vi "AddHelper.vi"() -> ()   [LabVIEW 2024, in "AddHelper.lvlib"]
uses:
  AddHelper.lvlib
  <vilib>/Utility/miscctls.llb/LVPointTypeDef.ctl
  <vilib>/Utility/traverseref.llb/TRef TravTarget.ctl
  <vilib>/event_ctls.llb/lveventtype.ctl
  templates/TemplateModule/TemplateModule.Start.vi
  templates/HelperTemplate.vi
  templates/TemplateModule/TemplateModule.lvclass
  <vilib>/Utility/traverseref.llb/VI Scripting - Traverse.lvlib
  <vilib>/Utility/Data Type/NI_Data Type.lvlib
panel:
  out "# of Refs 2":i32
  out "# of Refs":i32
  in  "Helper Name":string
  out "Child Type":refnum<vi>[](array[refnum])
  out "Same Type":refnum<vi>[](array[refnum])
  out "error out 2":errorcluster
  in  "Module Name":string
  out "Bottom":i32
  out "Left":i32
  out "error out":errorcluster
  in  "error in (no error)":errorcluster
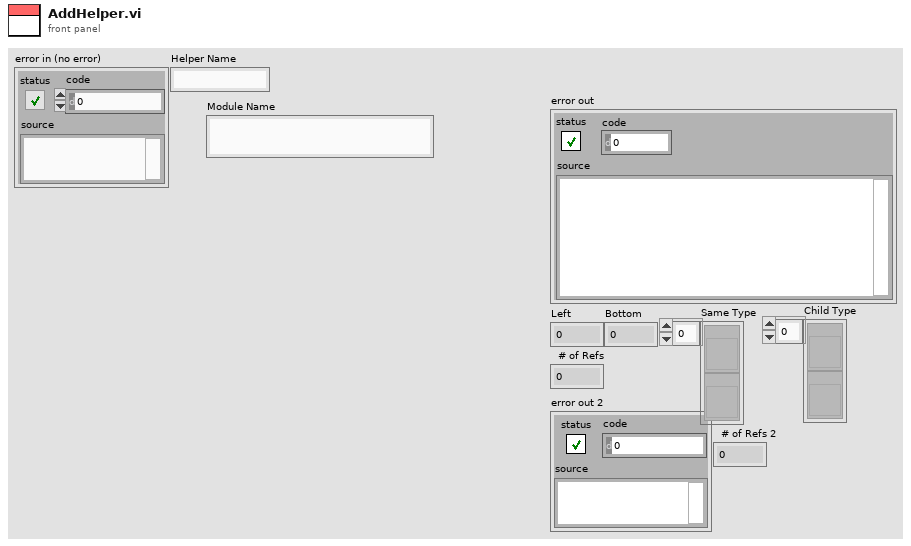
[diagram p1: front panel]
types:
  T1 = typedef "lveventtype.ctl" = enum32{"Null", "Timeout", "Annotation Menu Selection", "Annotation Menu Selection?", "App Instance Close", "App Instance Close?", "Autoscale Range Change", "Bookmark Info Change", "Cell Edit", "Cell Edit?", "Cursor Grab", "Cursor Grab?", "Cursor Menu Selection", "Cursor Menu Selection?", "Cursor Move", "Cursor Release", "Data Change", "Direction Change", "Display State Change", "Drag Ended", "Drag Enter", "Drag Leave", "Drag Over", "Drag Source Update", "Drag Starting", "Drag Starting?", "Drop", "Exec State Change", "Key Down", "Key Down?", "Key Repeat", "Key Repeat?", "Key Up", "Listbox Double Click", "Menu Activation?", "Menu Selection (App)", "Menu Selection? (App)", "Menu Selection (User)", "Mouse Down", "Mouse Down?", "Mouse Enter", "Mouse Leave", "Mouse Move", "Mouse Up", "Mouse Wheel", "NI Security User Change (App)", "Pane Size", "Panel Close", "Panel Close?", "Panel Resize", "Plot Attribute Change", "Scale Range Change", "Shortcut Menu Activation?", "Shortcut Menu Selection (App)", "Shortcut Menu Selection? (App)", "Shortcut Menu Selection (User)", "Tree Double Click", "Tree Drag", "Tree Drag?", "Tree Drop", "Tree Drop?", "Tree Item Close", "Tree Item Close?", "Tree Item Open", "Tree Item Open?", "User Event", "Value Change"}
  T2 = cluster{"Event Type":T1, "Event Registration Index":i32}[]
  T3 = typedef "TRef TravTarget.ctl" = enum16{"FP", "BD", "Other"}
  T4 = typedef "LVPointTypeDef.ctl" = cluster{"Horizontal":i16, "Vertical":i16}
  T5 = typedef "LVPositionTypeDef.ctl" = cluster{"Left":i32, "Top":i32}
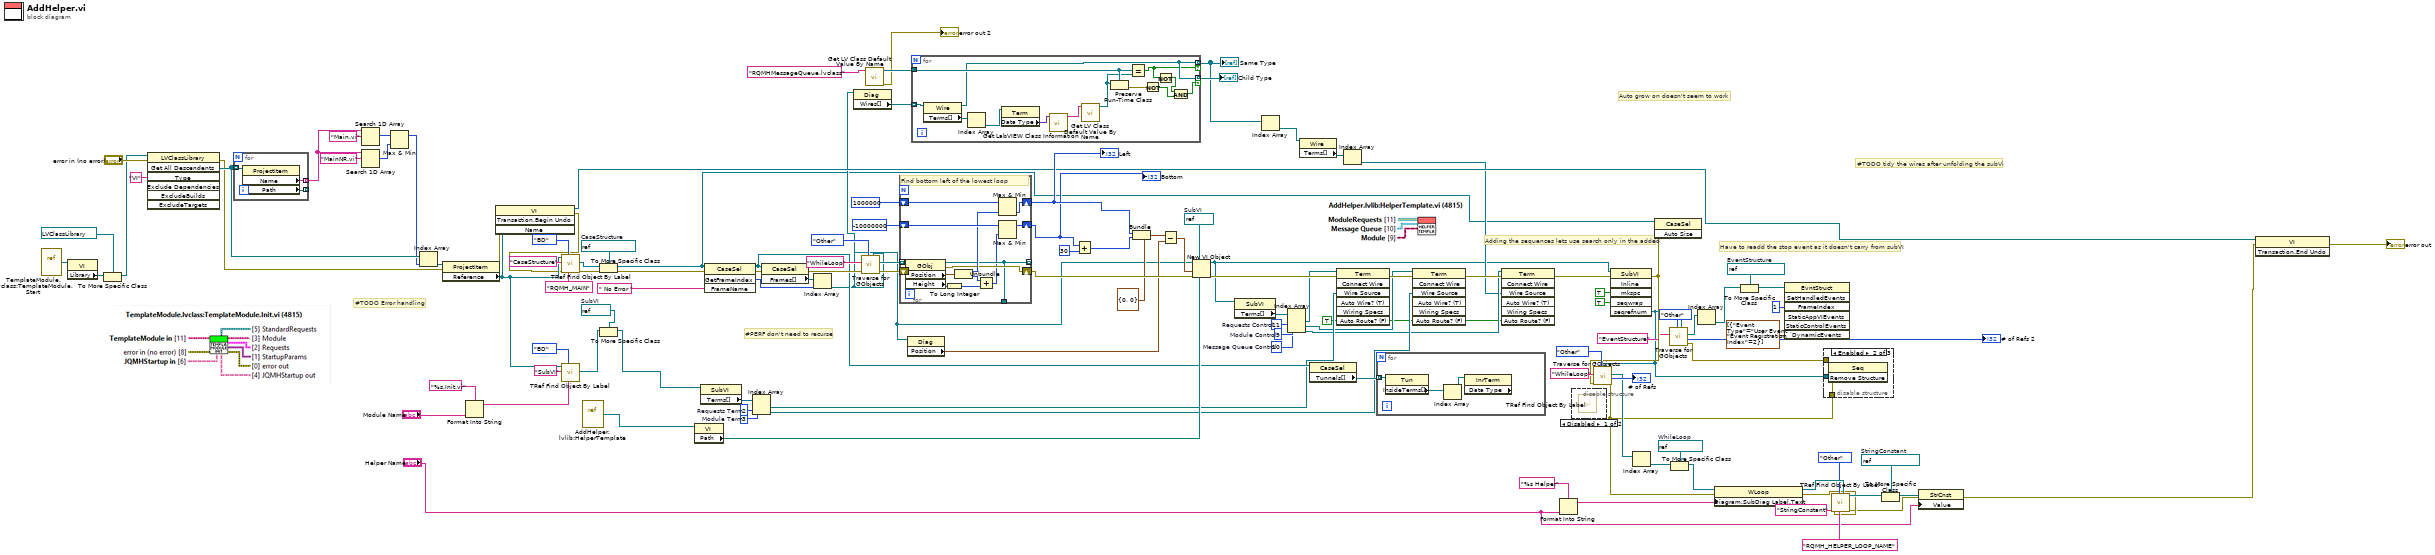
[diagram p0: block diagram]
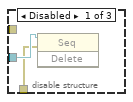
[diagram p2: hidden frame]
diagram:
  w7 = refnum<vi> refnum  # EventStructure
  w19 = refnum<vi> refnum  # StringConstant
  w30 = refnum<vi> refnum  # WhileLoop
  w58 = 10  # Message Queue Control
  w40 = TRUE ("Auto Route? (F)")
  w61 = 9  # Module Control
  w65 = 11  # Requests Control
  w67 = 3  # Module Term
  w68 = 2  # Requests Term
  w70 = refnum<vi> refnum  # SubVI
  w91 = refnum<vi> refnum  # SubVI
  w104 = refnum<vi> refnum  # CaseStructure
  # "Have to readd the stop event as it doesn't carry from subVI"
  # "#TODO tidy the wires after unfolding the subVi"
  # "Adding the sequences lets use search only in the added"
  # "Auto grow on doesn't seem to work"
  # "#PERF don't need to recurse"
  # "#TODO Error handling"
  n1 = vi-ref "TemplateModule.lvclass:TemplateModule.Start.vi"() -> (w110:refnum<vi>)
  n2 = property class="VI"(reference=w110) -> ("Library"=w108:refnum<vi>)  [unwired: 1 in, 2 out]
  n3 = To More Specific Class(target class=refnum<vi> refnum ("reference"), reference=w108) -> (specific class reference=w107:refnum<vi>)  [unwired: 1 in, 1 out]
  n4 = invoke class="LVClassLibrary" method="Get All Descendents"(reference=w107, error in="error in (no error)", "Type"="VI") -> (error out=w115:errorcluster, "All Descendents"=w118:refnum<vi>[])  [unwired: 4 in, 5 out]
  n5 = for {
    tunnel: w118 -> [w127] mode=indexing
    tunnel: [w126] -> w119 mode=indexing
    tunnel: [w125] -> _ mode=indexing
    n6 = property class="ProjectItem"(reference=w127) -> ("Name"=w126:string, "Path"=w125:path)  [unwired: 1 in, 2 out]
  }
  n7 = Search 1D Array(1D array=w119, element="Main.vi") -> (index of element=w121:i32)  [unwired: 1 in]
  n8 = Search 1D Array(1D array=w119, element="MainNR.vi") -> (index of element=w120:i32)  [unwired: 1 in]
  n9 = Max & Min(x=w121, y=w120) -> (max(x,y)=w116:i32)  [unwired: 1 out]
  n10 = Index Array(array=w118, index=w116) -> (element=w117:refnum<vi>)
  n11 = property class="ProjectItem"(reference=w117, error in=w115) -> (error out=w51:errorcluster, "Reference"=w52:refnum<vi>)  [unwired: 1 out]
  n12 = Format Into String(format string="%s.Init.vi", "Module Name") -> (resulting string=w75:string)  [unwired: 2 in, 1 out]
  n13 = invoke class="VI" method="Transaction.Begin Undo"(reference=w52, error in=w51) -> (reference out=w49:refnum<vi>, error out=w50:errorcluster)  [unwired: 2 in, 2 out]
  n14 = call <vilib>:"TRef Find Object By Label.vi"("Label"="RQMH_MAIN", "Traverse Target"=TRef_TravTarget."BD", "error in (no error)"=w50, "Class Name"="CaseStructure", "VI Ref"=w52) -> ("error out"=w106:errorcluster, "Found Obj Ref"=w105:refnum<vi>)  [unwired: 3 in, 2 out]
  n15 = call <vilib>:"TRef Find Object By Label.vi"("Label"=w75, "Traverse Target"=TRef_TravTarget."BD", "Class Name"="SubVI", "VI Ref"=w52) -> ("Found Obj Ref"=w72:refnum<vi>)  [unwired: 4 in, 3 out]
  n16 = vi-ref "AddHelper.lvlib:HelperTemplate.vi"() -> (w82:refnum<vi>)
  n17 = To More Specific Class(target class=w104, reference=w105, error in=w106) -> (specific class reference=w36:refnum<vi>, error out=w35:errorcluster)
  n18 = To More Specific Class(target class=w70, reference=w72) -> (specific class reference=w71:refnum<vi>)  [unwired: 1 in, 1 out]
  n19 = property class="VI"(reference=w82) -> ("Path"=w81:path)  [unwired: 1 in, 2 out]
  n20 = property class="SubVI"(reference=w71) -> ("Terms[]"=w69:refnum<vi>[])  [unwired: 1 in, 2 out]
  n21 = invoke class="CaseSel" method="GetFrameIndex"(reference=w36, error in=w35, "FrameName"=" No Error " ("Frame Name")) -> (reference out=w79:refnum<vi>, error out=w102:errorcluster, "GetFrameIndex"=w100:i32)  [unwired: 1 in, 1 out]
  n22 = Index Array(array=w69, index #1=w68, index #2=w67) -> (element #1=w63:refnum<vi>, element #2=w59:refnum<vi>)
  n23 = property class="CaseSel"(reference=w79, error in=w102) -> (error out=w99:errorcluster, "Frames[]"=w101:refnum<vi>[])  [unwired: 1 out]
  n24 = Index Array(array=w101, index=w100) -> (element=w47:refnum<vi>)
  n25 = property class="Diag"(reference=w47) -> ("Wires[]"=w46:refnum<vi>[])  [unwired: 1 in, 2 out]
  n26 = call <vilib>:"Traverse for GObjects.vi"("Other Refnum"=w47, "Traverse Target"=TRef_TravTarget."Other", "error in (no error)"=w99, "Class Name"="WhileLoop") -> ("error out"=w93:errorcluster, "References"=w96:refnum<vi>[])  [unwired: 4 in, 2 out]
  n27 = call <vilib>:"Get LV Class Default Value By Name.vi"("class name"="RQMHMessageQueue.lvclass") -> ("error out"=→"error out 2":errorcluster, "object"=w44:refnum<class>)  [unwired: 9 in]
  n28 = for {
    tunnel: w96 -> [w141] mode=indexing
    tunnel: [w133] -> _ mode=indexing
    shift-right: [w137] -> w86
    shift-left: 1000000 ("Left") -> [w139]
    shift-right: [w132] -> w85
    shift-left: -10000000 ("Left") -> [w138]
    shift-right: [w134] -> w92
    shift-left: w93 -> [w135]
    tunnel: [w133] -> _
    # "Find bottom left of the lowest loop"
    n29 = property class="GObj"(reference=w141, error in=w135) -> (reference out=w133:refnum<vi>, error out=w134:errorcluster, "Position"=w140:T5, "Height"=w130:u32)
    n30 = To Long Integer(number=w130) -> (32bit integer=w128:i32)
    n31 = Unbundle(w140) -> ("Left"=w136:i32, "Top"=w131:i32)
    n32 = Add(x=w131, y=w128) -> (x+y=w129:i32)
    n33 = Max & Min(x=w139, y=w136) -> (min(x,y)=w137:i32)  [unwired: 1 out]
    n34 = Max & Min(x=w138, y=w129) -> (max(x,y)=w132:i32)  [unwired: 1 out]
  }
  "Left" <- w86
  "Bottom" <- w85
  n35 = property class="Diag"(reference=w47) -> ("Position"=w88:T5)  [unwired: 1 in, 2 out]
  n36 = for {
    tunnel: w46 -> [w154] mode=indexing
    tunnel: w44 -> [w148]
    tunnel: [w146] -> w41 mode=indexing if=w145
    tunnel: [w146] -> w42 mode=indexing if=w142
    n37 = property class="Wire"(reference=w154) -> (reference out=w146:refnum<vi>, "Terms[]"=w153:refnum<vi>[])  [unwired: 1 in, 1 out]
    n38 = Index Array(array=w153) -> (element=w152:refnum<vi>)  [unwired: 1 in]
    n39 = property class="Term"(reference=w152) -> ("Data Type"=w151:variant)  [unwired: 1 in, 2 out]
    n40 = call <vilib>:"Get LabVIEW Class Information.vi"("variant"=w151) -> ("LabVIEW class file name"=w150:string)  [unwired: 8 in, 2 out]
    n41 = call <vilib>:"Get LV Class Default Value By Name.vi"("class name"=w150) -> ("object"=w147:refnum<class>)  [unwired: 9 in, 1 out]
    n42 = Preserve Run-Time Class(object in=w147, 2:w148) -> (error out=w149:errorcluster)  [unwired: 1 in, 1 out]
    n43 = Equal?(x=w148, y=w147) -> (x = y?=w145:bool)
    n44 = Not(x=w149) -> (.not. x?=w144:bool)
    n45 = Not(x=w145) -> (.not. x?=w143:bool)
    n46 = And(x=w143, y=w144) -> (x .and. y?=w142:bool)
  }
  "Same Type" <- w41
  "Child Type" <- w42
  n47 = Add(x=w85, y=30) -> (x+y=w83:i32)
  n48 = Bundle(cluster=T4 {"Horizontal"=0, "Vertical"=0} ("location"), "Horizontal"=w86, "Vertical"=w83) -> (w89:T4)
  n49 = Subtract(x=w89, y=w88) -> (x-y=w87:T5)
  n50 = New VI Object(vi object class=w91, owner refnum=w47, position/next to=w87, 6:w81, 8:w92) -> (object refnum=w34:refnum<vi>, 0:w80:errorcluster)  [unwired: 3 in]
  n51 = property class="SubVI"(reference=w34) -> ("Terms[]"=w66:refnum<vi>[])  [unwired: 1 in, 2 out]
  n52 = Index Array(array=w41) -> (element=w38:refnum<vi>)  [unwired: 1 in]
  n53 = Index Array(array=w66, index #1=w65, index #2=w61, index #3=w58) -> (element #1=w64:refnum<vi>, element #2=w60:refnum<vi>, element #3=w54:refnum<vi>)
  n54 = property class="Wire"(reference=w38) -> ("Terms[]"=w39:refnum<vi>[])  [unwired: 1 in, 2 out]
  n55 = property class="CaseSel"(reference=w79) -> ("Tunnels[]"=w78:refnum<vi>[])  [unwired: 1 in, 2 out]
  n56 = invoke class="Term" method="Connect Wire"(reference=w64, error in=w80, "Wire Source"=w63, "Auto Route? (F)"=w40) -> (error out=w62:errorcluster)  [unwired: 3 in, 6 out]
  n57 = Index Array(array=w39) -> (element=w37:refnum<vi>)  [unwired: 1 in]
  n58 = for {
    tunnel: w78 -> [w157] mode=indexing
    n59 = property class="Tun"(reference=w157) -> ("InsideTerms[]"=w156:refnum<vi>[])  [unwired: 1 in, 2 out]
    n60 = Index Array(array=w156) -> (element=w155:refnum<vi>)  [unwired: 1 in]
    n61 = property class="InrTerm" props=["Data Type"](reference=w155) -> ()  [unwired: 1 in, 3 out]
  }
  n62 = invoke class="Term" method="Connect Wire"(reference=w60, error in=w62, "Wire Source"=w59, "Auto Route? (F)"=w40) -> (error out=w55:errorcluster)  [unwired: 3 in, 6 out]
  n63 = invoke class="Term" method="Connect Wire"(reference=w54, error in=w55, "Wire Source"=w37, "Auto Route? (F)"=w40) -> (error out=w53:errorcluster)  [unwired: 3 in, 6 out]
  n64 = Format Into String(format string="%s Helper", "Helper Name") -> (resulting string=w25:string)  [unwired: 2 in, 1 out]
  n65 = disable-structure shown="Disabled" {
    frame Disabled {
      n66 = call <vilib>:"TRef Find Object By Label.vi"() -> ()  [unwired: 8 in, 4 out]
    }
    frame Enabled {
    }
  }
  n67 = invoke class="SubVI" method="Inline"(reference=w34, error in=w53, "mkspc"=TRUE ("Make Space in Block Diagram"), "seqwrap"=TRUE ("Wrap in Sequence")) -> (error out=w12:errorcluster, "seqrefnum"=w10:refnum<vi>)  [unwired: 2 in, 4 out]
  n68 = call <vilib>:"Traverse for GObjects.vi"("Other Refnum"=w10, "Traverse Target"=TRef_TravTarget."Other", "error in (no error)"=w12, "Class Name"="WhileLoop") -> ("error out"=w13:errorcluster, "# of Refs"=→"# of Refs":i32, "References"=w29:refnum<vi>[])  [unwired: 4 in, 1 out]
  n69 = Index Array(array=w29) -> (element=w28:refnum<vi>)  [unwired: 1 in]
  n70 = invoke class="CaseSel" method="Auto Size"(reference=w36, error in=w12) -> ()  [unwired: 1 in, 3 out]
  n71 = call <vilib>:"Traverse for GObjects.vi"("Other Refnum"=w10, "Traverse Target"=TRef_TravTarget."Other", "Class Name"="EventStructure") -> ("error out"=w8:errorcluster, "# of Refs"=→"# of Refs 2":i32, "References"=w2:refnum<vi>[])  [unwired: 5 in, 1 out]
  n72 = To More Specific Class(target class=w30, reference=w28) -> (specific class reference=w27:refnum<vi>)  [unwired: 1 in, 1 out]
  n73 = Index Array(array=w2) -> (element=w1:refnum<vi>)  [unwired: 1 in]
  n74 = property class="WLoop"(reference=w27, error in=w13, "Diagram.SubDiag Label.Text"=w25) -> (reference out=w23:refnum<vi>, error out=w16:errorcluster)
  n75 = To More Specific Class(target class=w7, reference=w1) -> (specific class reference=w6:refnum<vi>)  [unwired: 1 in, 1 out]
  n76 = invoke class="EvntStruct" method="SetHandledEvents"(reference=w6, "FrameIndex"=1 ("Frame Index"), "DynamicEvents"=T2 [{"Event Type"=enum."User Event", "Event Registration Index"=2}] ("Dynamic Events")) -> ()  [unwired: 4 in, 7 out]
  n77 = disable-structure shown="Enabled" {
    disable-tunnel: w10 -> [w159 w161 _]
    disable-tunnel: w13 -> [w158 w160 _]
    disable-tunnel: w8 -> [_ _ _]
    frame Disabled {
      n78 = invoke class="Seq" method="Delete"(reference=w159, error in=w158) -> ()  [unwired: 1 in, 3 out]
    }
    frame Enabled {
      n79 = invoke class="Seq" method="Remove Structure"(reference=w161, error in=w160) -> ()  [unwired: 1 in, 3 out]
    }
    frame Disabled {
    }
  }
  n80 = call <vilib>:"TRef Find Object By Label.vi"("Other Refnum"=w23, "Label"="RQMH_HELPER_LOOP_NAME", "Traverse Target"=TRef_TravTarget."Other", "error in (no error)"=w16, "Class Name"="StringConstant") -> ("error out"=w15:errorcluster, "dup VI Ref"=w20:refnum<vi>)  [unwired: 3 in, 2 out]
  n81 = To More Specific Class(target class=w19, reference=w20) -> (specific class reference=w18:refnum<vi>)  [unwired: 1 in, 1 out]
  n82 = property class="StrCnst"(reference=w18, error in=w15, "Value"="Helper Name") -> (error out=w14:errorcluster)  [unwired: 1 out]
  n83 = invoke class="VI" method="Transaction.End Undo"(reference=w49, error in=w14) -> (error out=→"error out":errorcluster)  [unwired: 1 in, 2 out]
